vi "SetVoltagGlobal.vi"() -> ()   [LabVIEW 2018]
panel:
  in  "SetVoltage":dbl
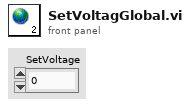
[diagram p1: front panel]
diagram:
